vi "Lim_DestroyPicture.vi"(8 "error in (no error)":errorcluster, 10 "LIMPICTURE":T2, 11 "hFile in":T1) -> (0 "error out":errorcluster, 3 "hFile out":T1)   [LabVIEW 2014, in "ND2_Reader_32.lvlib"]
doc: "This VI releases the Memory Space used for processing frames from the ND2 file."
uses:
  ND2_Reader_32.lvlib
  controls/cluster_LIMPICTURE.ctl
  controls/numeric_LIMFILEHANDLE.ctl
  nd2 reader/SDK/bin/x86/v6_w32_nd2ReadSDK.dll
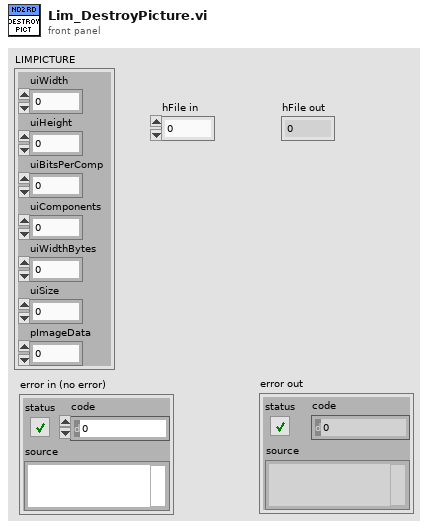
[diagram p1: front panel]
types:
  T1 = typedef "numeric_LIMFILEHANDLE.ctl" = i32
  T2 = typedef "cluster_LIMPICTURE.ctl" = cluster{"uiWidth":u32, "uiHeight":u32, "uiBitsPerComp":u32, "uiComponents":u32, "uiWidthBytes":u32, "uiSize":u32, "pImageData":u32}
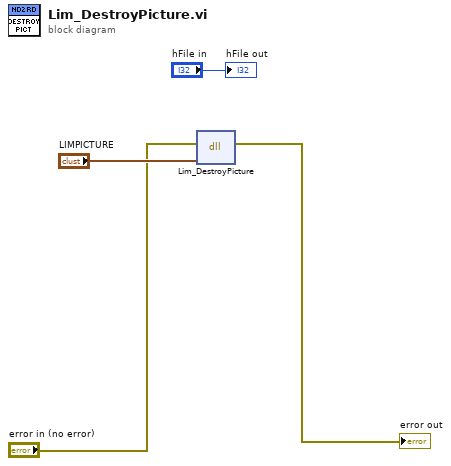
[diagram p0: block diagram]
diagram:
  n1 = dll-call lib="C:/Users/VirtualUser/Desktop/EPA-Vision/EPA Image Source LV2014 2.0.0 2016-02-23/ND2_Reader_32bit/nd2 reader/SDK/bin/x86/v6_w32_nd2ReadSDK.dll" fn="Lim_DestroyPicture"(error in="error in (no error)", "pPicture"="LIMPICTURE") -> (error out=→"error out":errorcluster)  [unwired: 2 in, 3 out]
  "hFile out" <- "hFile in"
